vi "Test Source VI.vi"(9 "B":dbl, 10 "A":dbl) -> (1 "A>B?":bool, 2 "sum":dbl)   [LabVIEW 2016]
panel:
  in  "Path":path
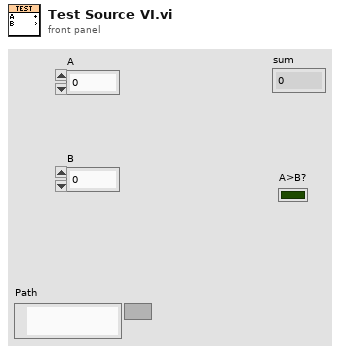
[diagram p1: front panel]
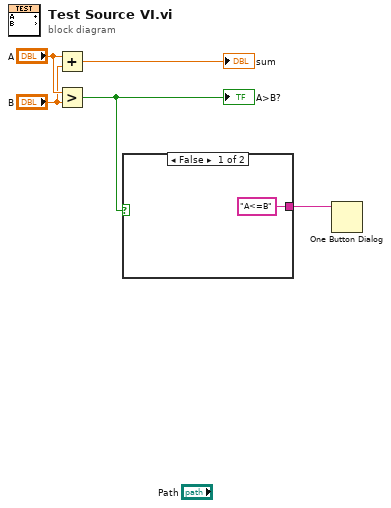
[diagram p0: block diagram]
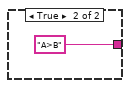
[diagram p2: hidden frame]
diagram:
  n1 = Add(x="A", y="B") -> (x+y=→"sum":dbl)
  n2 = Greater?(x="A", y="B") -> (0:w2:bool)
  "A>B?" <- w2
  n3 = case shown="False" w2 {
    tunnel: ["A<=B" ("message") "A>B" ("message")] -> w1
    frame False {
    }
    frame True {
    }
  }
  n4 = One Button Dialog(message=w1) -> ()  [unwired: 1 in, 1 out]
